vi "Vision Processing V.5.0.vi"(8 "error in (no error)":errorcluster, 11 "Image Size":T1=enum."320x240") -> ()   [LabVIEW 2016]
uses:
  Vision Support Code/Camera Types.ctl
  <vilib>/Rock Robotics/WPI/Camera/WPI_CameraImageSize.ctl
  <vilib>/Rock Robotics/WPI/Camera/WPI_CameraWhite Balance Values.ctl
  <vilib>/Rock Robotics/WPI/Camera/WPI_CameraFrameRate.ctl
  <vilib>/Rock Robotics/WPI/Camera/WPI_CameraExposure Values.ctl
  Robot Global Data V.5.0.vi
  <vilib>/Rock Robotics/Network Tables/NT Write Number.vi
  <vilib>/vision/NI_Vision_Development_Module.lvlib
panel:
  out "loop ms":u32
  out "Calibration error":errorcluster
  in  "Display Original":bool
  in  "Display Mask":bool
  in  "Line Border":cluster{"Top":dbl, "Bottom":dbl}={"Top"=6.0, "Bottom"=1.0}
  in  "Use Calibration":bool=TRUE
  out "Instructions:":string="Use Source to load image files from a directory, or use a USB or IP camera connected to your laptop. Use Camera Settings 1 and 2 to achieve a dark image with bright and colorful stripes.\nLED Color can encoded as HSL or related color modes. Calibrate to the same color as the strips being reflected to the camera.\nClick and draw a line in Original Image to auto-calibrate the LED Color. You may want to widen and tweak Sat and Val by hand.\nThe Annotate button affects drawing a rectangle around the stripes and labeling it with a distance in ft. Distance relies on knowing the Camera Type and lens calibration (it looks up the lens view angle).\n\nAdjust Score Cutoff to make the code more or less picky. If the color is not very unique, you may need to increase the number of particles considered. The diagram uses a Size Limit to ignore colored things that are too small. You may need to adjust it if you are targetting from far away.\n\nResults give you the distance to the target, the center and box in a normalized (-1 to 1) and pixel coordinates.\n\nBe sure to read about setting camera exposure and brightness to help simplify your image and acquire color saturated images.\n\nThere are lots of comments on the diagram to explain the code."
  in  "Color Mode":u16(ring)=3 items=["RGB", "HSL", "HSV", "HSI"]
  in  "Particles":dbl=5.0
  in  "Score Cutoff %":dbl=70.0
  in  "Camera Type":T2=enum."MS HD3000 square"
  out "Results":T3 {"Score" format="%#_3g"; "Pixels"."Rectangle"."Numeric 5" format="%#_3g"; "Pixels"."Rectangle"."Numeric 3" format="%#_3g"; "Pixels"."Rectangle"."Numeric 2" format="%#_3g"; "Pixels"."Rectangle"."Numeric" format="%#_3g"; "Normalized"."Rectangle"."Numeric 5" format="%#_2g"; "Normalized"."Rectangle"."Numeric 3" format="%#_2g"; "Normalized"."Rectangle"."Numeric 2" format="%#_2g"; "Normalized"."Rectangle"."Numeric" format="%#_2g"; "Normalized"."Center"."?" format="%#_3g"; "Normalized"."Center"."?" format="%#_3g"; "Distance (ft)" format="%#_3g"}
  out "Qualified Particles":i32
  in  "LED Color":T4={"Hue"={107.81818389892578, 139.81818389892578}, "Sat"={176.07142857142858, 255.0}, "Val"={40.53571428571429, 255.0}} {"Hue" scale=0.0..255.0 scale format="%#_3g"}
  out "Mask":T5(plugin-control)
  out "Original Image":T5(plugin-control)
  # "Legend:\n    Rectangle\n       Green - Good target, distance ft\n       Red - Bad target\n    Orange Text - Score in %"
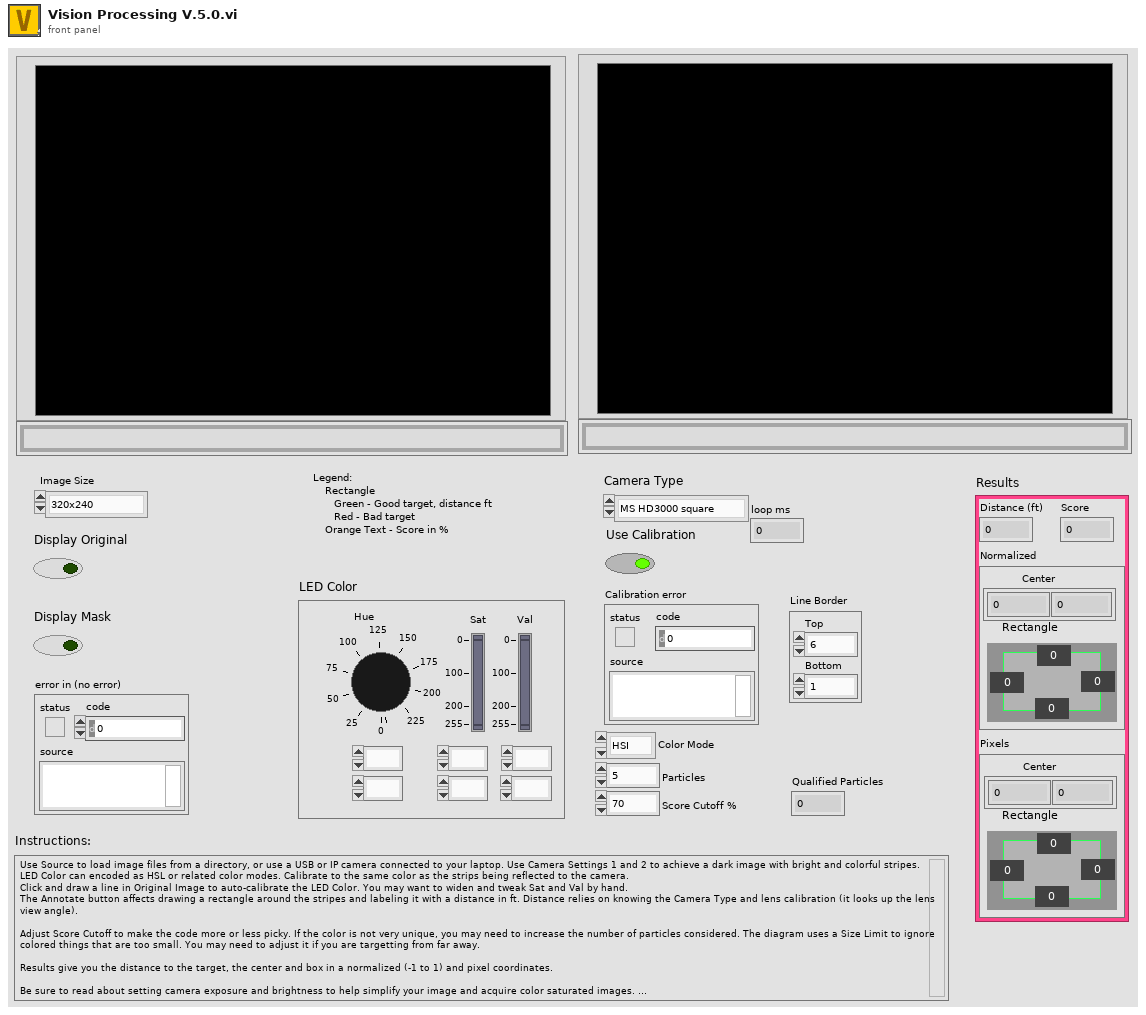
[diagram p1: front panel]
types:
  T1 = typedef "WPI_CameraImageSize.ctl" = enum16{"640x480", "320x240", "160x120", "Custom"}
  T2 = typedef "Camera Types.ctl" = enum16{"206", "1011", "1013", "MS HD3000 square", "MS HD3000 640x480"}
  T3 = cluster{"Distance (ft)":dbl, "Score":dbl, "Normalized":cluster{"Center":cluster{dbl, dbl}, "Rectangle":cluster{"Numeric":dbl, "Numeric 2":dbl, "Numeric 3":dbl, "Numeric 5":dbl}}, "Pixels":cluster{"Center":cluster{dbl, dbl}, "Rectangle":cluster{"Numeric":dbl, "Numeric 2":dbl, "Numeric 3":dbl, "Numeric 5":dbl}}}
  T4 = cluster{"Hue":cluster{dbl, dbl}, "Sat":cluster{dbl, dbl}, "Val":cluster{dbl, dbl}}
  T5 = typedef "IMAQ Image.ctl" = refnum<image>
  T6 = typedef "WPI_CameraFrameRate.ctl" = u32
  T7 = typedef "WPI_CameraWhite Balance Values.ctl" = enum16{"Auto", "Fixed indoor", "Fixed outdoor 1", "Fixed outdoor 2", "Fixed fluorescent 1", "Fixed fluorescent 2", "Hold current", "Custom"}
  T8 = typedef "Image Type" = u32
  T9 = typedef "Particle Parameters" = i32
  T10 = typedef "WPI_CameraDevRef.ctl" = cluster{"Camera Address":string, "CameraStatus":errorcluster}
  T11 = typedef "WPI_CameraExposure Values.ctl" = enum16{"Auto", "Flicker-free 50 Hz", "Flicker-free 60 Hz", "Hold current", "Custom"}
  T12 = cluster{"Left":dbl, "Top":dbl, "Right":dbl, "Bottom":dbl}
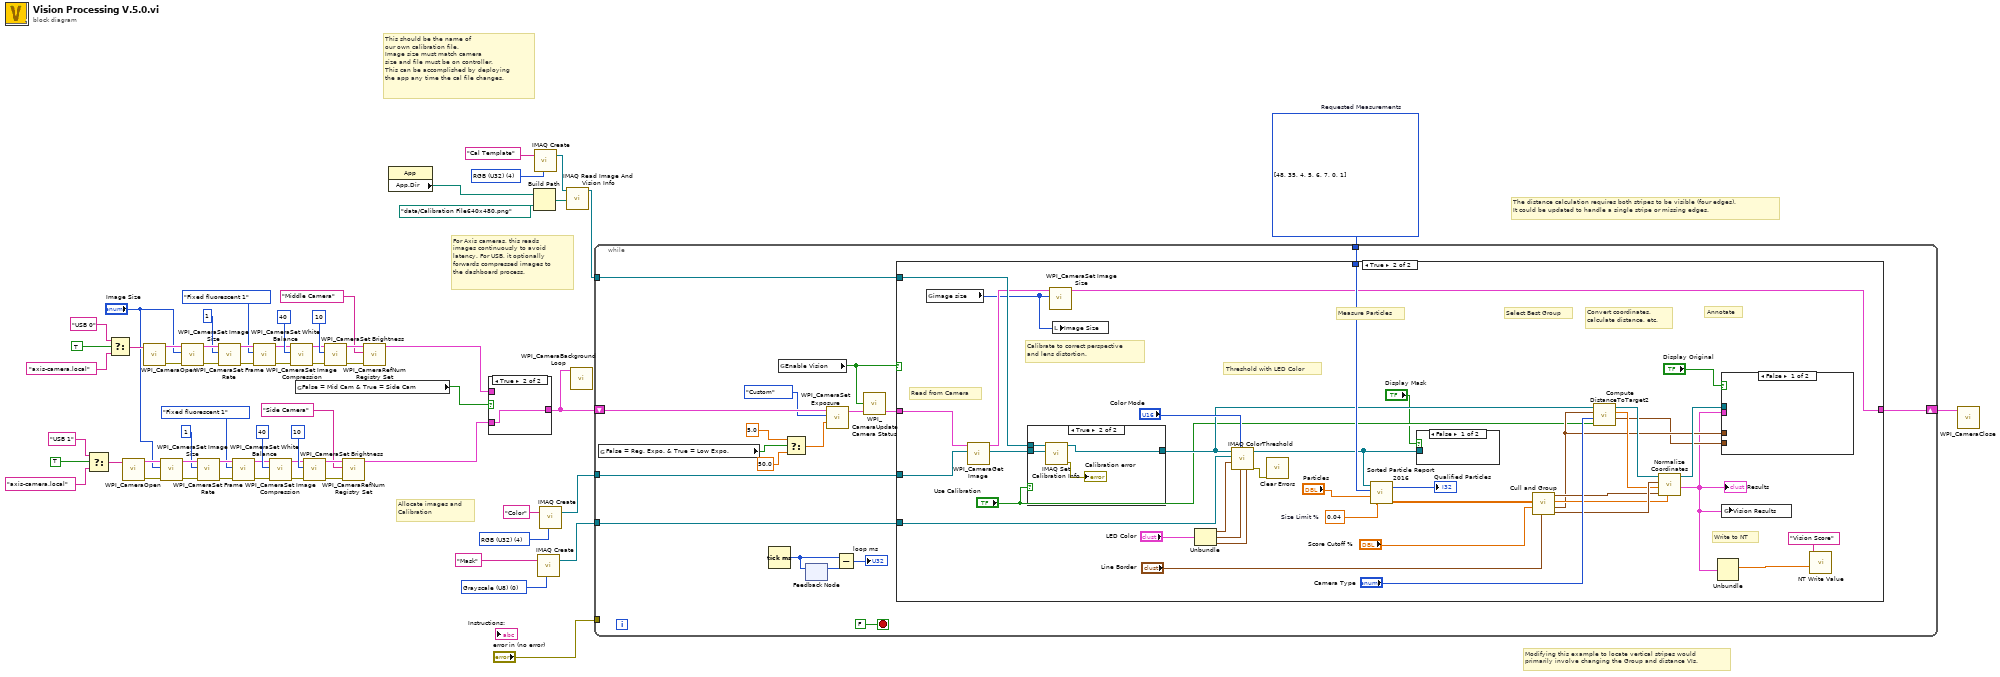
[diagram p0: block diagram]
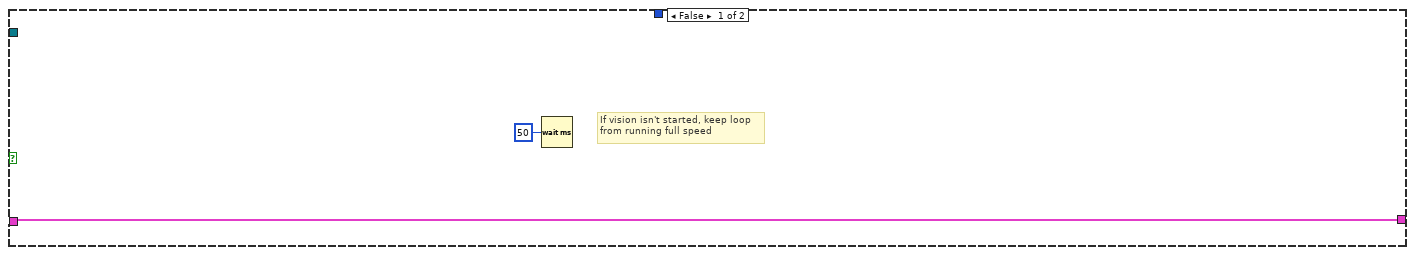
[diagram p3: hidden frame]
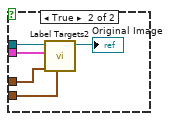
[diagram p4: hidden frame]
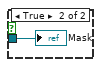
[diagram p5: hidden frame]
diagram:
  w56 = T8 4 items=["Grayscale (U8)", "Grayscale (I16)", "Grayscale (SGL)", "Complex (CSG)", "RGB (U32)", "HSL (U32)", "RGB (U64)", "Grayscale (U16)"] ("Image Type")
  w58 = T9[] [48, 35, 4, 5, 6, 7, 0, 1] items=["Center of Mass X", "Center of Mass Y", "First Pixel X", "First Pixel Y", "Bounding Rect Left", "Bounding Rect Top", "Bounding Rect Right", "Bounding Rect Bottom", "Max Feret Diameter Start X", "Max Feret Diameter Start Y", "Max Feret Diameter End X", "Max Feret Diameter End Y", "Max Horiz. Segment Length Left", "Max Horiz. Segment Length Right", "Max Horiz. Segment Length Row", "-", "Bounding Rect Width", "Bounding Rect Height", "Bounding Rect Diagonal", "Perimeter", "Convex Hull Perimeter", "Holes' Perimeter", "Max Feret Diameter", "Equivalent Ellipse Major Axis", "Equivalent Ellipse Minor Axis", "Equivalent Ellipse Minor Axis (Feret)", "Equivalent Rect Long Side", "Equivalent Rect Short Side", "Equivalent Rect Diagonal", "Equivalent Rect Short Side (Feret)", "Average Horiz. Segment Length", "Average Vert. Segment Length", "Hydraulic Radius", "Waddel Disk Diameter", "-", "Area", "Holes' Area", "Particle & Holes' Area", "Convex Hull Area", "Image Area", "-", "Number of Holes", "Number of Horiz. Segments", "Number of Vert. Segments", "-", "Orientation", "Max Feret Diameter Orientation", "-", "% Area/Image Area", "% Area/(Particle & Holes' Area)", "Ratio of Equivalent Ellipse Axes", "Ratio of Equivalent Rect Sides", "-", "Elongation Factor", "Compactness Factor", "Heywood Circularity Factor", "Type Factor", "-", "Sum X", "Sum Y", "Sum XX", "Sum XY", "Sum YY", "Sum XXX", "Sum XXY", "Sum XYY", "Sum YYY", "-", "Moment of Inertia XX", "Moment of Inertia XY", "Moment of Inertia YY", "Moment of Inertia XXX", "Moment of Inertia XXY", "Moment of Inertia XYY", "Moment of Inertia YYY", "Norm. Moment of Inertia XX", "Norm. Moment of Inertia XY", "Norm. Moment of Inertia YY", "Norm. Moment of Inertia XXX", "Norm. Moment of Inertia XXY", "Norm. Moment of Inertia XYY", "Norm. Moment of Inertia YYY", "Hu Moment 1", "Hu Moment 2", "Hu Moment 3", "Hu Moment 4", "Hu Moment 5", "Hu Moment 6", "Hu Moment 7"]  # Requested Measurements
  w61 = T8 0 items=["Grayscale (U8)", "Grayscale (I16)", "Grayscale (SGL)", "Complex (CSG)", "RGB (U32)", "HSL (U32)", "RGB (U64)", "Grayscale (U16)"] ("Image Type")
  w62 = T8 4 items=["Grayscale (U8)", "Grayscale (I16)", "Grayscale (SGL)", "Complex (CSG)", "RGB (U32)", "HSL (U32)", "RGB (U64)", "Grayscale (U16)"] ("Image Type")
  # "This should be the name of \nour own calibration file.\nImage size must match camera\nsize and file must be on controller.\nThis can be accomplished by deploying\nthe app any time the cal file changes."
  # "For Axis cameras, this reads\nimages continuously to avoid\nlatency. For USB, it optionally\nforwards compressed images to\nthe dashboard process."
  # "Modifying this example to locate vertical stripes would\nprimarily involve changing the Group and distance VIs."
  # "The distance calculation requires both stripes to be visible (four edges).\nIt could be updated to handle a single stripe or missing edges."
  # "Allocate images and\nCalibration"
  n1 = Select(t="USB 1" ("format string"), s=TRUE ("dot notation? (F)"), f="axis-camera.local" ("format string")) -> (s? t:f=w7:string)
  n2 = Select(t="USB 0" ("format string"), s=TRUE ("dot notation? (F)"), f="axis-camera.local" ("format string")) -> (s? t:f=w33:string)
  n3 = call <vilib>:"WPI_CameraOpen.vi"("Camera Address"=w7) -> ("error out"=w16:errorcluster, "CameraDevRef"=w17:T10)  [unwired: 1 in, 8 out]
  n4 = call <vilib>:"WPI_CameraOpen.vi"("Camera Address"=w33) -> ("error out"=w42:errorcluster, "CameraDevRef"=w43:T10)  [unwired: 1 in, 8 out]
  n5 = call <vilib>:"WPI_CameraSet Image Size.vi"("error in (no error)"=w16, "Image Size"="Image Size", "CameraDevRef"=w17) -> ("error out"=w15:errorcluster, "CameraDevRef Out"=w18:T10)  [unwired: 1 in, 6 out]
  n6 = call <vilib>:"WPI_CameraSet Image Size.vi"("error in (no error)"=w42, "Image Size"="Image Size", "CameraDevRef"=w43) -> ("error out"=w41:errorcluster, "CameraDevRef Out"=w44:T10)  [unwired: 1 in, 6 out]
  n7 = call <vilib>:"WPI_CameraSet Frame Rate.vi"("error in (no error)"=w15, "Frame Rate (fps)"=T6 1, "CameraDevRef"=w18) -> ("error out"=w14:errorcluster, "CameraDevRef Out"=w19:T10)  [unwired: 7 out]
  n8 = call <vilib>:"WPI_CameraSet Frame Rate.vi"("error in (no error)"=w41, "Frame Rate (fps)"=T6 1, "CameraDevRef"=w44) -> ("error out"=w40:errorcluster, "CameraDevRef Out"=w45:T10)  [unwired: 7 out]
  n9 = call <vilib>:"WPI_CameraSet White Balance.vi"("error in (no error)"=w14, "White Balance"=WPI_CameraWhite_Balance_Values."Fixed fluorescent 1", "CameraDevRef"=w19) -> ("error out"=w5:errorcluster, "CameraDevRef Out"=w6:T10)  [unwired: 1 in, 6 out]
  n10 = call <vilib>:"WPI_CameraSet White Balance.vi"("error in (no error)"=w40, "White Balance"=WPI_CameraWhite_Balance_Values."Fixed fluorescent 1", "CameraDevRef"=w45) -> ("error out"=w28:errorcluster, "CameraDevRef Out"=w29:T10)  [unwired: 1 in, 6 out]
  n11 = call <vilib>:"WPI_CameraSet Image Compression.vi"("error in (no error)"=w5, "Compression"=40, "CameraDevRef"=w6) -> ("error out"=w13:errorcluster, "CameraDevRef Out"=w20:T10)  [unwired: 7 out]
  n12 = call <vilib>:"WPI_CameraSet Image Compression.vi"("error in (no error)"=w28, "Compression"=40, "CameraDevRef"=w29) -> ("error out"=w39:errorcluster, "CameraDevRef Out"=w46:T10)  [unwired: 7 out]
  n13 = global read "Robot Global Data V.5.0.vi" "False = Mid Cam & True = Side Cam"() -> (w2:bool)
  n14 = call <vilib>:"WPI_CameraSet Brightness.vi"("error in (no error)"=w13, "Brightness"=10, "CameraDevRef"=w20) -> ("error out"=w12:errorcluster, "CameraDevRef Out"=w24:T10)  [unwired: 7 out]
  n15 = call <vilib>:"WPI_CameraSet Brightness.vi"("error in (no error)"=w39, "Brightness"=10, "CameraDevRef"=w46) -> ("error out"=w38:errorcluster, "CameraDevRef Out"=w50:T10)  [unwired: 7 out]
  n16 = call <vilib>:"WPI_CameraRefNum Registry Set.vi"("error in (no error)"=w12, "refnum name"="Side Camera", "CameraDevRef"=w24) -> ("CameraDevRef"=w3:T10)  [unwired: 1 in, 7 out]
  n17 = call <vilib>:"WPI_CameraRefNum Registry Set.vi"("error in (no error)"=w38, "refnum name"="Middle Camera", "CameraDevRef"=w50) -> ("CameraDevRef"=w26:T10)  [unwired: 1 in, 7 out]
  n18 = property class="App"() -> ("App.Dir"=w30:path)  [unwired: 2 in, 2 out]
  n19 = case shown="True" w2 {
    tunnel: [w64 w65] -> w25
    tunnel: w26 -> [w64 _]
    tunnel: w3 -> [_ w65]
    frame False {
    }
    frame True {
    }
  }
  n20 = Build Path(base path=w30, name or relative path=path "data/Calibration File640x480.png" ("Folder Location")) -> (appended path=w52:path)
  n21 = call "IMAQ Create"("Image Name"="Cal Template", "Image Type"=w56) -> ("New Image"=w54:T5)  [unwired: 2 in, 2 out]
  n22 = call "IMAQ Create"("Image Name"="Mask", "Image Type"=w61) -> ("New Image"=w59:T5)  [unwired: 2 in, 2 out]
  n23 = call "IMAQ Create"("Image Name"="Color", "Image Type"=w62) -> ("New Image"=w57:T5)  [unwired: 2 in, 2 out]
  n24 = call "IMAQ Read Image And Vision Info"("File Path"=w52, "Image"=w54) -> ("Image Out"=w53:T5)  [unwired: 7 in, 2 out]
  n25 = call <vilib>:"WPI_CameraBackground Loop.vi"("CameraDevRef"=w25) -> ()  [unwired: 11 in]
  n26 = while {
    tunnel: w57 -> [w79]
    tunnel: w59 -> [w82]
    tunnel: w58 -> [w81]
    tunnel: w53 -> [w80]
    shift-right: [w78] -> w32
    shift-left: w25 -> [w71]
    tunnel: "error in (no error)" -> [_]
    stop <- FALSE stop-if-true
    n27 = global read "Robot Global Data V.5.0.vi" "False = Reg. Expo. & True = Low Expo."() -> (w67:bool)
    n28 = Tick Count (ms)() -> (millisecond timer value=w74:u32)
    n29 = global read "Robot Global Data V.5.0.vi" "Enable Vision"() -> (w76:bool)
    n30 = Select(t=5.0, s=w67, f=50.0) -> (s? t:f=w66:dbl)
    n31 = feedback-in #1(w74) -> ()
    n32 = feedback #1() -> (w75:u32)  [unwired: 1 in]
    n33 = call <vilib>:"WPI_CameraSet Exposure.vi"("Exposure (%)"=w66, "Exposure"=WPI_CameraExposure_Values."Custom", "CameraDevRef"=w71) -> ("CameraDevRef Out"=w72:T10)  [unwired: 1 in, 7 out]
    n34 = Subtract(x=w74, y=w75) -> (x-y=→"loop ms":u32)
    n35 = call <vilib>:"WPI_CameraUpdate Camera Status.vi"("CameraDevRef In"=w72, "Enable Vision"=w76) -> ("CameraDevRef Out"=w77:T10)  [unwired: 3 in]
    n36 = case shown="True" w76 {
      tunnel: w82 -> [_ w123]
      tunnel: w81 -> [_ w119]
      tunnel: w80 -> [_ w99]
      tunnel: w77 -> [w85 w96]
      tunnel: w79 -> [_ w95]
      tunnel: [w85 w90] -> w78
      frame False {
        # "If vision isn't started, keep loop\nfrom running full speed"
        n37 = Wait (ms)(milliseconds to wait=u32 50) -> ()  [unwired: 1 out]
      }
      frame True {
        w117 = 0.04  # Size Limit %
        # "Write to NT"
        # "Read from Camera"
        # "Calibrate to correct perspective\nand lens distortion."
        # "Measure Particles"
        # "Convert coordinates,\ncalculate distance, etc."
        # "Annotate"
        # "Select Best Group"
        # "Threshold with LED Color"
        n38 = global read "Robot Global Data V.5.0.vi" "image size"() -> (w89:T1)
        n39 = call <vilib>:"WPI_CameraGet Image.vi"("Image"=w95, "CameraDevRef"=w96) -> ("Image Out"=w94:T5, "CameraDevRef Out"=w91:T10)  [unwired: 7 in, 1 out]
        n40 = case shown="True" "Use Calibration" {
          tunnel: [w130 w134] -> w100
          tunnel: w94 -> [w130 w133]
          tunnel: w99 -> [_ w132]
          frame False {
          }
          frame True {
            n41 = call "IMAQ Set Calibration Info"("Image Dst"=w133, "Image Src"=w132) -> ("error out"=→"Calibration error":errorcluster, "Calibrated Image"=w134:T5)  [unwired: 8 in]
          }
        }
        n42 = call <vilib>:"WPI_CameraSet Image Size.vi"("Image Size"=w89, "CameraDevRef"=w91) -> ("CameraDevRef Out"=w90:T10)  [unwired: 2 in, 7 out]
        n43 = local write "Image Size"(w89) -> ()
        n44 = Unbundle("LED Color") -> ("Hue"=w122:cluster{dbl, dbl}, "Sat"=w121:cluster{dbl, dbl}, "Val"=w120:cluster{dbl, dbl})
        n45 = call "IMAQ ColorThreshold"("Blue or Luma or Val or Inten Range"=w120, "Green or Sat Range"=w121, "Color Mode"="Color Mode", "Red or Hue Range"=w122, "Image Dst"=w123, "Image Src"=w100) -> ("error out"=w116:errorcluster, "Image Dst Out"=w112:T5)  [unwired: 4 in]
        n46 = call <vilib>:"Clear Errors.vi"("error in (no error)"=w116) -> ()  [unwired: 5 in, 2 out]
        n47 = call "Sorted Particle Report 2016.vi"("Min Area Size %"=w117, "Particle Count Limit"="Particles", "Pixel Measurements"=w119, "Image in"=w112) -> ("Sorted Data"=w114:dbl[][], "Particles"=→"Qualified Particles":i32)
        n48 = case shown="False" "Display Mask" {
          tunnel: w112 -> [_ w129]
          frame False {
          }
          frame True {
            "Mask" <- w129
          }
        }
        n49 = call "Cull and Group.vi"("Line Border"="Line Border", "Score Cutoff"="Score Cutoff %", "Sorted Data"=w114) -> ("Rect"=w110:T12, "Line"=w102:T12, "Score"=w105:dbl, "Center"=w106:cluster{"X":dbl, "Y":dbl})  [unwired: 5 in]
        n50 = call "Compute DistanceToTarget2.vi"("Calibrated"="Use Calibration", "Camera Type"="Camera Type", "Line"=w102, "Image Src"=w100) -> ("Edges"=w101:cluster{"X":sgl, "Y":sgl}[], "Distance (ft)"=w109:dbl, "Image Dst Out"=w108:T5)  [unwired: 5 in]
        n51 = call "Normalize Coordinates.vi"("Score"=w105, "Center"=w106, "Distance"=w109, "Bounding box"=w110, "Image in"=w108) -> ("Results"=w88:T3, "Image out"=w107:T5)  [unwired: 5 in]
        "Results" <- w88
        n52 = Unbundle(w88) -> ("Score"=w87:dbl)  [unwired: 3 out]
        n53 = case shown="False" "Display Original" {
          tunnel: w107 -> [_ w127]
          tunnel: w88 -> [_ w126]
          tunnel: w102 -> [_ w125]
          tunnel: w101 -> [_ w124]
          frame False {
          }
          frame True {
            n54 = call "Label Targets2.vi"("Edges"=w124, "Line"=w125, "Results"=w126, "Image in"=w127) -> ("Image out"=→"Original Image":T5)  [unwired: 7 in]
          }
        }
        n55 = global write "Robot Global Data V.5.0.vi" "Vision Results"(w88) -> ()
        n56 = call-poly <vilib>:"NT Write Value.vi"("Numeric"=w87, "Name"="Vision Score") -> ()  [unwired: 9 in, 1 out]
      }
    }
  }
  n57 = call <vilib>:"WPI_CameraClose.vi"("CameraDevRef"=w32) -> ()  [unwired: 1 in, 10 out]
